vi "Run.vi"(8 "error in (no error)":errorcluster caption="entrée d'erreur (pas d'erreur)", 9 "Y":string[][](array[string]), 10 "X":string[][](array[string]), 11 "Sigmoid_kernel.lvclass":refnum<class "Sigmoid_kernel.lvclass">) -> (0 "error out":errorcluster caption="sortie d'erreur", 2 "Data":T1, 3 "Sigmoid_kernel.lvclass":refnum<class "Sigmoid_kernel.lvclass">)   [LabVIEW 2020, in "Sigmoid_kernel.lvclass"]
doc: "Returns :\n\n- Gram matrix : array of shape (n_samples_1, n_samples_2)"
uses:
  Sigmoid_kernel.lvclass
  Sigmoid_kernel.lvclass/Sigmoid_kernel.ctl
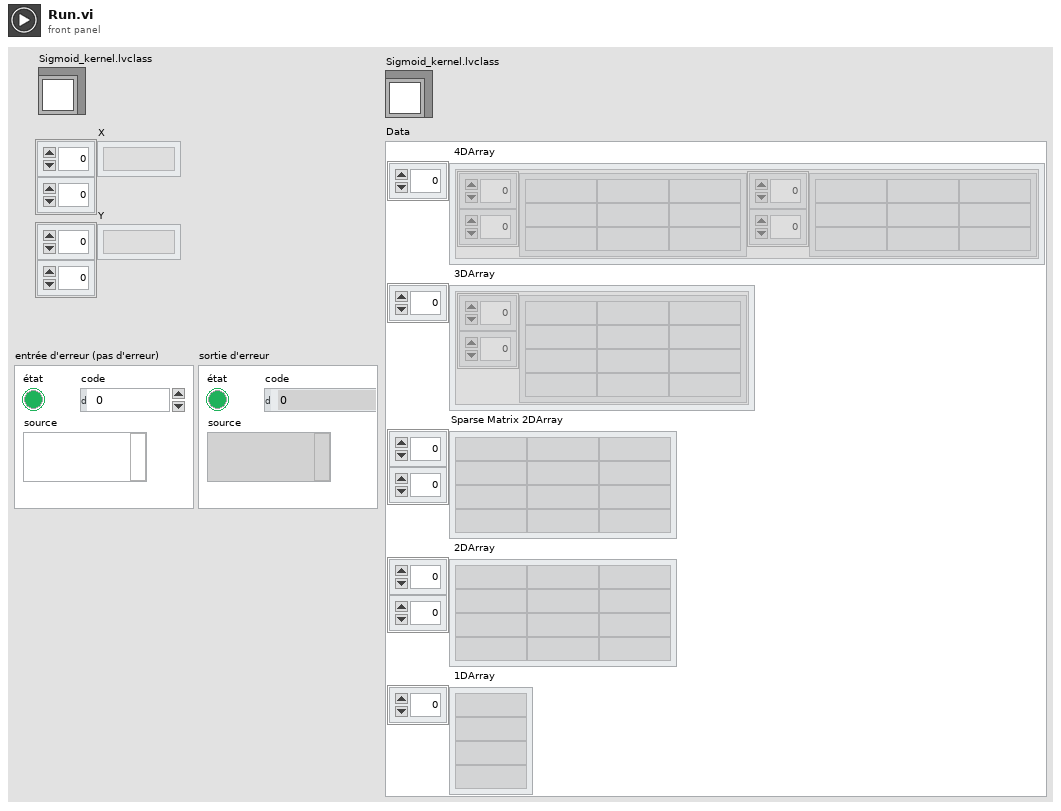
[diagram p1: front panel]
types:
  T1 = cluster{" 4DArray":cluster{"1":string[][], "2":string[][]}[], " 3DArray":cluster{"Tableau":string[][]}[], "Sparse Matrix 2DArray":string[][], " 2DArray":string[][], " 1DArray":string[]}
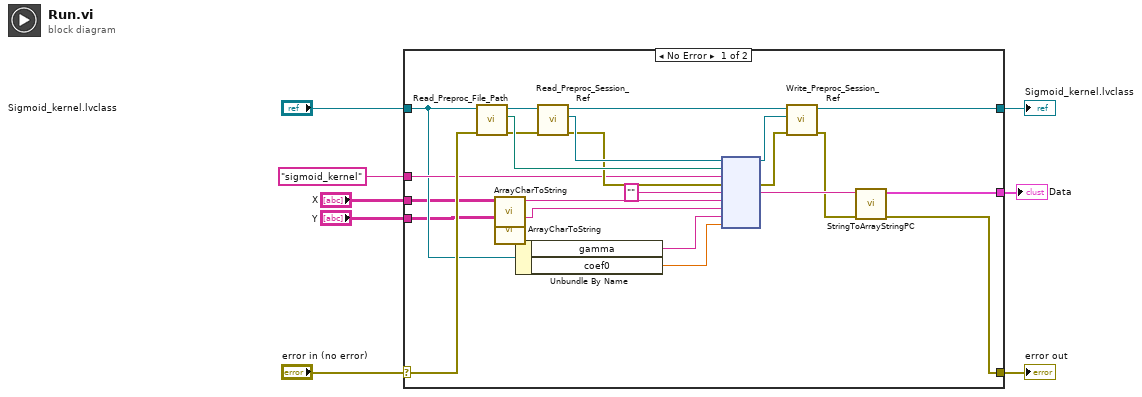
[diagram p0: block diagram]
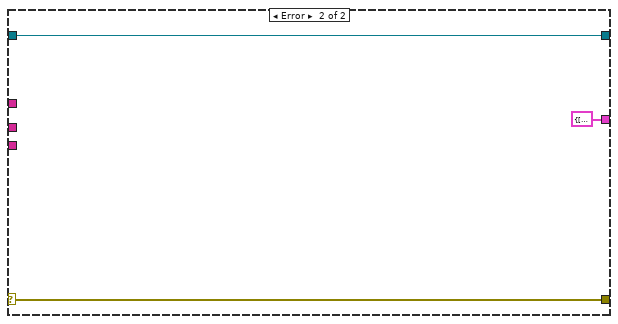
[diagram p2: hidden frame]
diagram:
  n1 = case shown="No Error" "error in (no error)" {
    selector: "error in (no error)" -> [w22 w34]
    tunnel: [w10 w34] -> w7
    tunnel: [w17 w33] -> w5
    tunnel: "Sigmoid_kernel.lvclass" -> [w20 w33]
    tunnel: "sigmoid_kernel" ("Fonction") -> [w21 _]
    tunnel: "X" -> [w16 _]
    tunnel: "Y" -> [w15 _]
    tunnel: [w9 T1 {" 4DArray"=[], " 3DArray"=[], "Sparse Matrix 2DArray"=[], " 2DArray"=[], " 1DArray"=[]} ("Data")] -> w1
    frame No Error {
      n2 = call-dynamic "Read_Preproc_File_Path.vi"("error in (no error)"=w22, "Python in"=w20) -> ("error out"=w26:errorcluster, "File_Path"=w29:path, "Python out"=w31:refnum<class "Sigmoid_kernel.lvclass">)  [unwired: 7 in]
      n3 = call "ArrayCharToString.vi"("TAB"=w16) -> ("Instruction"=w14:string)  [unwired: 10 in]
      n4 = call "ArrayCharToString.vi"("TAB"=w15) -> ("Instruction"=w13:string)  [unwired: 10 in]
      n5 = Unbundle By Name(w20) -> ("gamma"=w19:string, "coef0"=w18:dbl)
      n6 = call-dynamic "Read_Preproc_Session_Ref.vi"("error in (no error)"=w26, "Python in"=w31) -> ("error out"=w27:errorcluster, "Session_ref"=w28:refnum<k35>, "Python out"=w30:refnum<class "Sigmoid_kernel.lvclass">)  [unwired: 7 in]
      n7 = node(w28, w29, w21, w27, "", w14, w13, w19, w18) -> (w23:refnum<k35>, w25:errorcluster, w12:string)  [unwired: 4 in, 2 out]
      n8 = call-dynamic "Write_Preproc_Session_Ref.vi"("error in (no error)"=w25, "Session_ref"=w23, "Python in"=w30) -> ("error out"=w11:errorcluster, "Python out"=w17:refnum<class "Sigmoid_kernel.lvclass">)  [unwired: 7 in]
      n9 = call "StringToArrayStringPC.vi"("sortie d'erreur"=w11, "Return value"=w12) -> ("sortie d'erreur"=w10:errorcluster, "Data"=w9:T1)  [unwired: 8 in]
    }
    frame Error {
    }
  }
  "error out" <- w7
  "Sigmoid_kernel.lvclass" <- w5
  "Data" <- w1
